vi "Parse_SubVI.vi"(11 "SCPI String":string="COMmand:SUBcommand (1:2|0) PARameters") -> (0 "Channel_Array":i32[](array[numeric]), 1 "Device_Array":i32[](array[numeric]), 2 "SubCommand":string, 3 "Command":string, 4 "Parameters":string)   [LabVIEW 2021]
panel:
  out "Channel_List":string
  out "Device_List":string
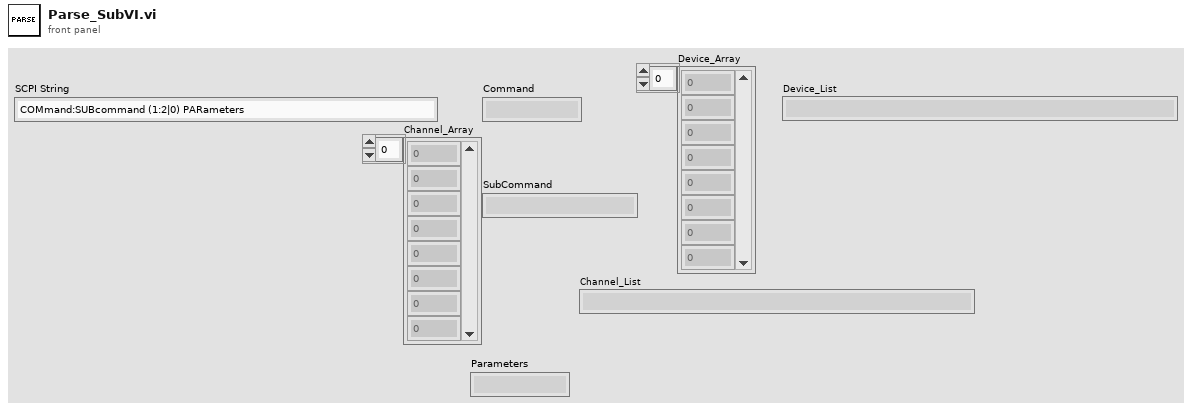
[diagram p1: front panel]
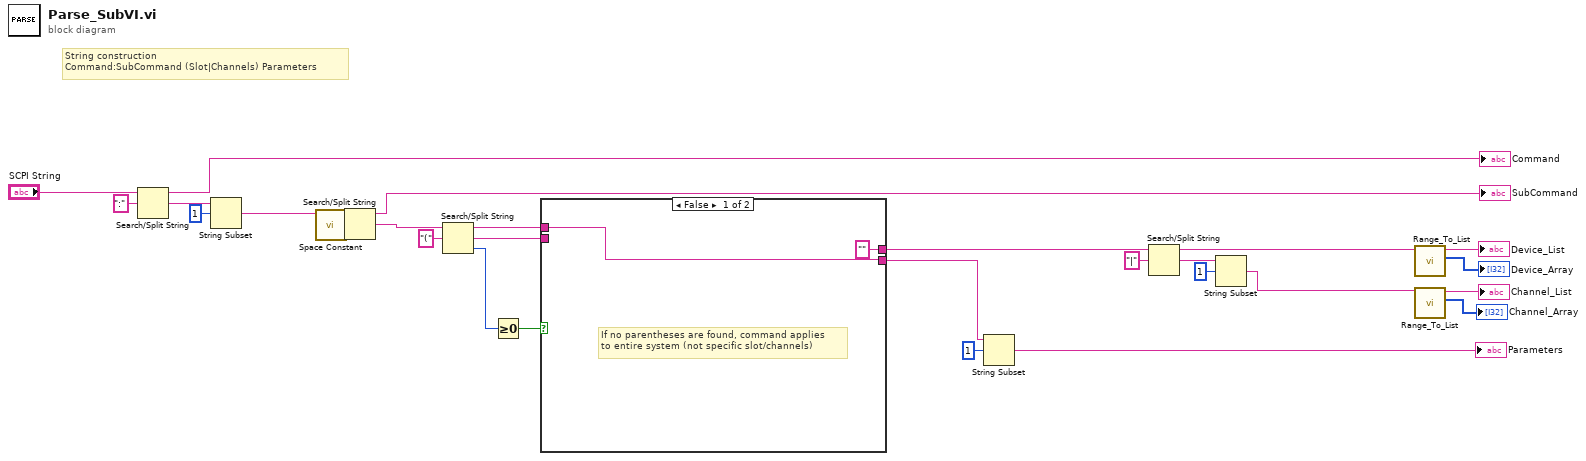
[diagram p0: block diagram]
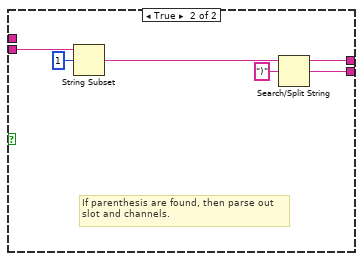
[diagram p2: hidden frame]
diagram:
  # "String construction\nCommand:SubCommand (Slot|Channels) Parameters"
  n1 = Search/Split String(string="SCPI String", search string/char (-)=":") -> (substring before match=→"Command":string, match + rest of string=w25:string)  [unwired: 1 in, 1 out]
  n2 = String Subset(string=w25, offset (0)=1) -> (substring=w12:string)  [unwired: 1 in]
  n3 = call <vilib>:"Space Constant.vi"() -> ("String"=w10:string)
  n4 = Search/Split String(string=w12, search string/char (-)=w10) -> (substring before match=→"SubCommand":string, match + rest of string=w9:string)  [unwired: 1 in, 1 out]
  n5 = Search/Split String(string=w9, search string/char (-)="(") -> (substring before match=w7:string, match + rest of string=w20:string, offset of match=w21:i32)  [unwired: 1 in]
  n6 = Greater Or Equal To 0?(x=w21) -> (x >= 0?=w8:bool)
  n7 = case shown="False" w8 {
    tunnel: w20 -> [_ w34]
    tunnel: [w28 w31] -> w18
    tunnel: ["" ("SCPI String") w30] -> w14
    tunnel: w7 -> [w28 _]
    frame False {
      # "If no parentheses are found, command applies\nto entire system (not specific slot/channels)"
    }
    frame True {
      # "If parenthesis are found, then parse out\nslot and channels."
      n8 = String Subset(string=w34, offset (0)=1) -> (substring=w33:string)  [unwired: 1 in]
      n9 = Search/Split String(string=w33, search string/char (-)=")") -> (substring before match=w30:string, match + rest of string=w31:string)  [unwired: 1 in, 1 out]
    }
  }
  n10 = String Subset(string=w18, offset (0)=1) -> (substring=→"Parameters":string)  [unwired: 1 in]
  n11 = Search/Split String(string=w14, search string/char (-)="|") -> (substring before match=w6:string, match + rest of string=w15:string)  [unwired: 1 in, 1 out]
  n12 = String Subset(string=w15, offset (0)=1) -> (substring=w3:string)  [unwired: 1 in]
  n13 = call "Range_To_List.vi"("Range String"=w6) -> ("Array"=→"Device_Array":i32[], "List"=→"Device_List":string)  [unwired: 9 in]
  n14 = call "Range_To_List.vi"("Range String"=w3) -> ("Array"=→"Channel_Array":i32[], "List"=→"Channel_List":string)  [unwired: 9 in]
